vi "Initialise.vi"(6 "Tag Root":string, 8 "error in (no error)":errorcluster, 9 "Update Rate (Hz) - Non HW Timed":dbl=10.0, 10 "timeout (s)":dbl=10.0, 11 "DAQmx Device":refnum<k21>) -> (0 "error out":errorcluster, 3 "DAQmx-Bus out":refnum<class "DAQmx-Bus.lvclass">)   [LabVIEW 2021, in "DAQmx-Bus.lvclass"]
uses:
  DAQmx-Bus.lvclass
  C:/Program Files (x86)/National Instruments/LabVIEW 2021/vi.lib/TSA/Omni-Bus/Omni-Bus/Bus Access/Bus_Access.lvclass
  Support/Task Handlers/Analog In Multi Sample/DAQmx - Analog Input Multi Sample.lvclass
  C:/TSA/DAQmx-Bus/Source/DAQmx-Bus.lvclass
  Support/Task Handlers/Analog In Single Sample/DAQmx - Analog Input Single Sample.lvclass
  Support/Task Handlers/Analog Out Multi Sample/DAQmx - Analog Output Multi Sample.lvclass
  Support/Task Handlers/Analog Out Single Sample/DAQmx - Analog Output Single Sample.lvclass
  Support/Task Handlers/Digital In Single Sample/DAQmx - Digital Input Single Sample.lvclass
  DAQmx-Bus.lvclass/DAQmx-Bus.ctl
  <vilib>/TSA/Omni-Bus/Omni-Bus/Bus Access/Bus_Access.lvclass/Bus_Access.ctl
  Properties/Write DAQmx Task.vi
  <vilib>/TSA/Omni-Bus/Omni-Bus/Bus Access/Properties/Write Tag Root.vi
  Properties/Write timeout.vi
  Properties/Write Update Rate.vi
  <resource>/objmgr/daqmx.rc
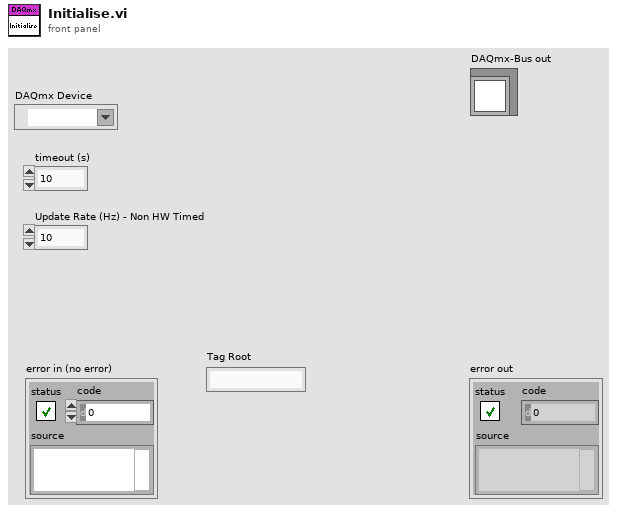
[diagram p1: front panel]
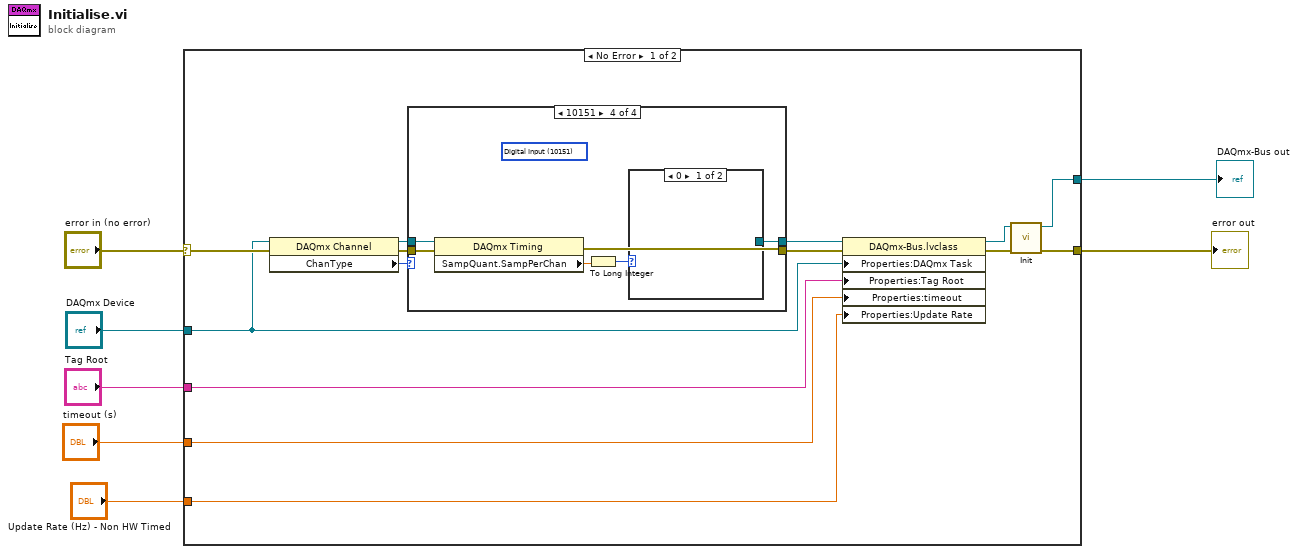
[diagram p0: block diagram]
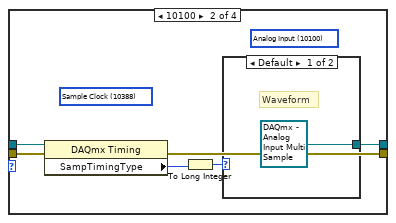
[diagram p3: hidden frame]
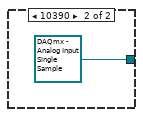
[diagram p4: hidden frame]
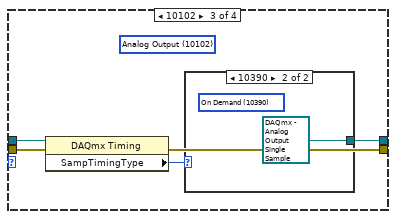
[diagram p5: hidden frame]
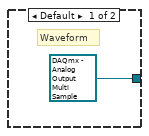
[diagram p6: hidden frame]
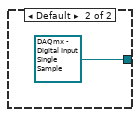
[diagram p7: hidden frame]
diagram:
  n1 = case shown="No Error" "error in (no error)" {
    selector: "error in (no error)" -> [w18 w45]
    tunnel: [w13 w45] -> w6
    tunnel: [w12 _] -> w5
    tunnel: "DAQmx Device" -> [w9 _]
    tunnel: "Tag Root" -> [w17 _]
    tunnel: "timeout (s)" -> [w19 _]
    tunnel: "Update Rate (Hz) - Non HW Timed" -> [w10 _]
    frame No Error {
      n2 = property class="DAQmx Channel"(reference=w9, error in=w18) -> (reference out=w8:refnum<k21>, error out=w20:errorcluster, "ChanType"=w21:i32)
      n3 = case shown="10151" w21 {
        tunnel: w20 -> [w22 w27 w33 w41]
        tunnel: [_ w28 w35 w43] -> w15
        tunnel: [w22 w25 w31 w39] -> w16
        tunnel: w8 -> [_ w26 w34 w40]
        frame Default {
        }
        frame 10100 {
          (unwired) 10388 items=["Sample Clock"=10388, "Burst Handshake"=12548, "Handshake"=10389, "Implicit"=10451, "On Demand"=10390, "Change Detection"=12504, "Pipelined Sample Clock"=14668] ("SampTimingType")
          (unwired) 10100 items=["Analog Input"=10100, "Analog Output"=10102, "Digital Input"=10151, "Digital Output"=10153, "Counter Input"=10131, "Counter Output"=10132] ("ChanType")
          n4 = property class="DAQmx Timing"(reference=w26, error in=w27) -> (error out=w25:errorcluster, "SampTimingType"=w24:i32)  [unwired: 1 out]
          n5 = To Long Integer(number=w24) -> (32bit integer=w23:i32)
          n6 = case shown="Default" w23 {
            tunnel: [refnum<class "DAQmx - Analog Input Multi Sample.lvclass"> refnum ("DAQmx - Analog Input Multi Sample.lvclass") refnum<class "DAQmx - Analog Input Single Sample.lvclass"> refnum ("DAQmx - Analog Input Single Sample.lvclass")] -> w28
            frame Default {
              # "Waveform"
            }
            frame 10390 {
            }
          }
        }
        frame 10102 {
          (unwired) 10102 items=["Analog Input"=10100, "Analog Output"=10102, "Digital Input"=10151, "Digital Output"=10153, "Counter Input"=10131, "Counter Output"=10132] ("ChanType")
          n7 = property class="DAQmx Timing"(reference=w34, error in=w33) -> (error out=w31:errorcluster, "SampTimingType"=w32:i32)  [unwired: 1 out]
          n8 = case shown="10390" w32 {
            tunnel: [refnum<class "DAQmx - Analog Output Multi Sample.lvclass"> refnum ("DAQmx - Analog Output Multi Sample.lvclass") refnum<class "DAQmx - Analog Output Single Sample.lvclass"> refnum ("DAQmx - Analog Output Single Sample.lvclass")] -> w35
            frame Default {
              # "Waveform"
            }
            frame 10390 {
              (unwired) 10390 items=["Sample Clock"=10388, "Burst Handshake"=12548, "Handshake"=10389, "Implicit"=10451, "On Demand"=10390, "Change Detection"=12504, "Pipelined Sample Clock"=14668] ("SampTimingType")
            }
          }
        }
        frame 10151 {
          (unwired) 10151 items=["Analog Input"=10100, "Analog Output"=10102, "Digital Input"=10151, "Digital Output"=10153, "Counter Input"=10131, "Counter Output"=10132] ("ChanType")
          n9 = property class="DAQmx Timing"(reference=w40, error in=w41) -> (error out=w39:errorcluster, "SampQuant.SampPerChan"=w42:dbl)  [unwired: 1 out]
          n10 = To Long Integer(number=w42) -> (32bit integer=w38:i32)
          n11 = case shown="0" w38 {
            tunnel: [_ refnum<class "DAQmx - Digital Input Single Sample.lvclass"> refnum ("DAQmx - Digital Input Single Sample.lvclass")] -> w43
            frame 0 {
            }
            frame Default {
            }
          }
        }
      }
      n12 = property class="DAQmx-Bus.lvclass"(reference=w15, error in=w16, "Properties:DAQmx Task"=w9, "Properties:Tag Root"=w17, "Properties:timeout"=w19, "Properties:Update Rate"=w10) -> (reference out=w11:refnum<class "DAQmx-Bus.lvclass">, error out=w14:errorcluster)
      n13 = call-dynamic "Init.vi"("error in (no error)"=w14, "Data in"=w11) -> ("error out"=w13:errorcluster, "Data out"=w12:refnum<class "DAQmx-Bus.lvclass">)  [unwired: 8 in]
    }
    frame Error {
    }
  }
  "error out" <- w6
  "DAQmx-Bus out" <- w5
